vi "Measure_DUT_Current.vi"(8 "error in":errorcluster) -> (0 "error out":errorcluster, 3 "DUTCurrent":dbl)   [LabVIEW 2020]
panel:
  out "data":string
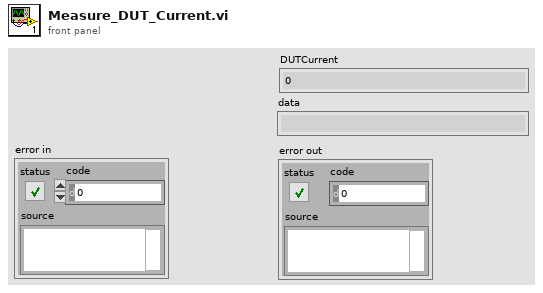
[diagram p1: front panel]
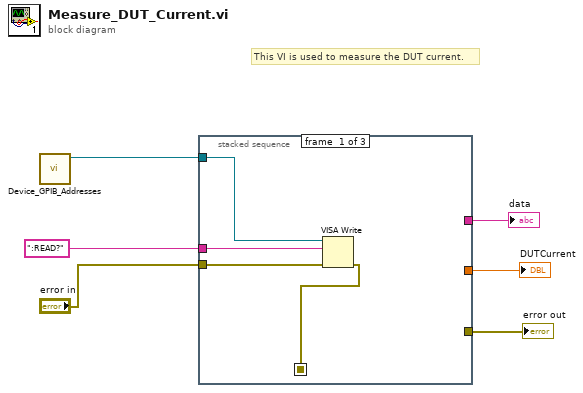
[diagram p0: block diagram]
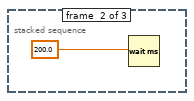
[diagram p2: hidden frame]
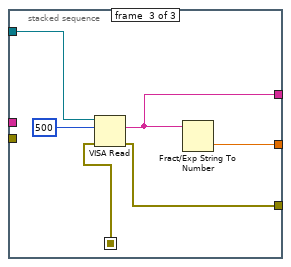
[diagram p3: hidden frame]
diagram:
  # "This VI is used to measure the DUT current."
  n1 = call "Device_GPIB_Addresses.vi"() -> ("Keithley 2400 Address"=w2:refnum<visa-resource-name>)  [unwired: 9 in, 2 out]
  n2 = stacked-sequence {
    seq-local: [w7 _ _] -> [_ _ w13]
    tunnel: ":READ?" -> [w9 _ _]
    tunnel: "error in" -> [w8 _ _]
    tunnel: [_ _ w17] -> w5
    tunnel: [_ _ w12] -> w4
    tunnel: [_ _ w16] -> w3
    tunnel: w2 -> [w10 _ w15]
    frame #0 {
      n3 = VISA Write(VISA resource name=w10, write buffer=w9, error in (no error)=w8) -> (error out=w7:errorcluster)  [unwired: 2 out]
    }
    frame #1 {
      n4 = Wait (ms)(milliseconds to wait=200.0) -> ()  [unwired: 1 out]
    }
    frame #2 {
      n5 = VISA Read(VISA resource name=w15, byte count=500, error in (no error)=w13) -> (read buffer=w16:string, error out=w12:errorcluster)  [unwired: 2 out]
      n6 = Fract/Exp String To Number(string=w16) -> (number=w17:dbl)  [unwired: 3 in, 1 out]
    }
  }
  "DUTCurrent" <- w5
  "error out" <- w4
  "data" <- w3
